vi "Write Multiple System Link Tags.vi"(7 "Force Initialize?":bool, 8 "error in (no error)":errorcluster, 9 "timestamp":timestamp, 10 "Values":dbl[](array[numeric]), 11 "SkyLine.Refs":refnum<class "NI Skyline Tag.lvclass">[](array[class])) -> (0 "error out":errorcluster)   [LabVIEW 2019, in "Data Publishing Service.lvlib"]
uses:
  Data Publishing Service.lvlib
  <vilib>/Skyline/Tag/Wrapper/Wrapper_class/NI Skyline Tag.lvclass
  <vilib>/Skyline/Tag/Wrapper/Wrapper_class/Tag Value Cluster Wrapper.ctl
  <vilib>/Skyline/Configuration/Configuration_class/NI Skyline Configuration.lvclass
  <vilib>/Skyline/Tag/Shared/typedefs/Tag Value Cluster.ctl
  <vilib>/Skyline/Tag/Shared/typedefs/DataType.ctl
  <vilib>/Skyline/Tag/Wrapper/Wrapper_class/Generate Tag Cluster (DBL) 2.vi
  <vilib>/Skyline/Tag/Shared/NI Skyline Tag.lvlib
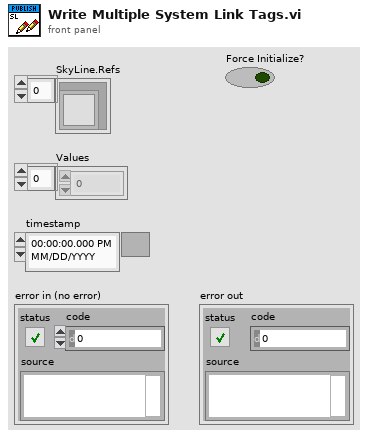
[diagram p1: front panel]
types:
  T1 = typedef "NI Skyline Tag.lvclass/Tag Value Cluster Wrapper.ctl" = cluster{"Configuration":refnum<class "NI Skyline Configuration.lvclass">, "Tag Cluster":T2}
  T2 = typedef "NI Skyline Tag.lvlib/Tag Value Cluster.ctl" = cluster{"Path":string, "Data Type":T3, "Value":string, "Time Stamp":timestamp}
  T3 = typedef "NI Skyline Tag.lvlib/DataType.ctl" = enum32{"Double", "I32", "String", "Boolean", "U64", "Timestamp"}
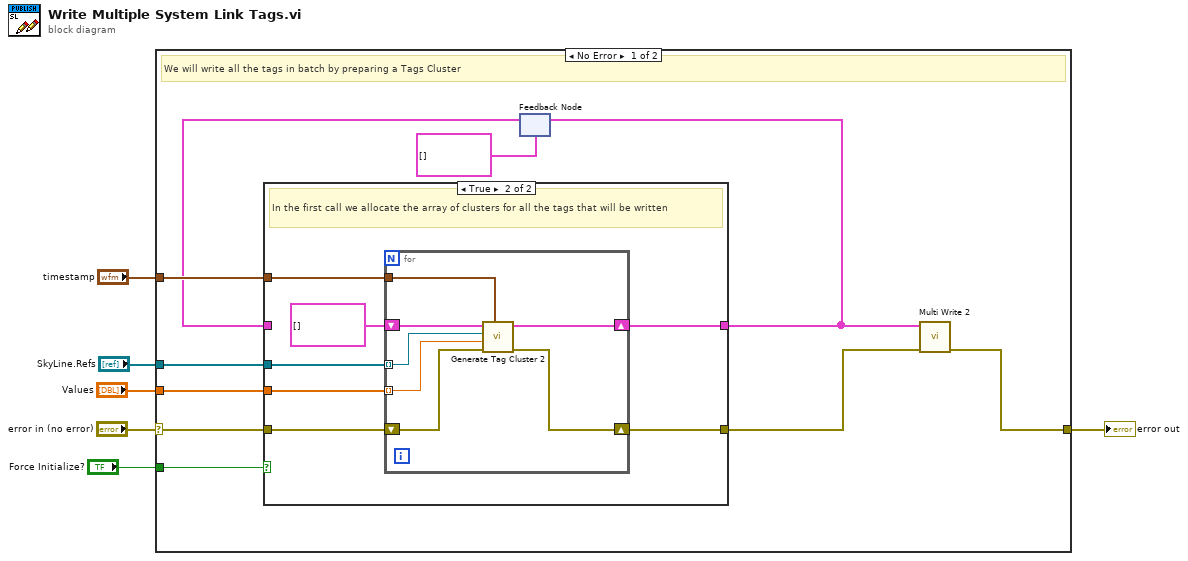
[diagram p0: block diagram]
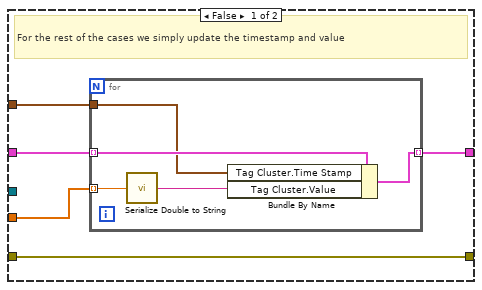
[diagram p2: hidden frame]
diagram:
  n1 = case shown="No Error" "error in (no error)" {
    selector: "error in (no error)" -> [w9 w41]
    tunnel: "SkyLine.Refs" -> [w16 _]
    tunnel: "Values" -> [w15 _]
    tunnel: "timestamp" -> [w14 _]
    tunnel: [w8 w41] -> w2
    tunnel: "Force Initialize?" -> [w7 _]
    frame No Error {
      # "We will write all the tags in batch by preparing a Tags Cluster"
      n2 = feedback #1(T1[] [] ("tag clusters in")) -> (w12:T1[])
      n3 = case shown="True" w7 {
        tunnel: w16 -> [_ w33]
        tunnel: w15 -> [w17 w32]
        tunnel: w9 -> [w21 w31]
        tunnel: w14 -> [w18 w30]
        tunnel: [w21 w29] -> w10
        tunnel: [w19 w28] -> w11
        tunnel: w12 -> [w20 _]
        frame False {
          # "For the rest of the cases we simply update the timestamp and value"
          n4 = for {
            tunnel: w20 -> [w26] mode=indexing
            tunnel: [w25] -> w19 mode=indexing
            tunnel: w18 -> [w24]
            tunnel: w17 -> [w22] mode=indexing
            n5 = call <vilib>:"Serialize Double to String.vi"("double"=w22) -> ("string"=w23:string)
            n6 = Bundle By Name(cluster=w26, "Tag Cluster.Time Stamp"=w24, "Tag Cluster.Value"=w23) -> (w25:T1)
          }
        }
        frame True {
          # "In the first call we allocate the array of clusters for all the tags that will be written"
          n7 = for {
            shift-right: [w36] -> w28
            shift-left: T1[] [] ("tag clusters in") -> [w40]
            tunnel: w33 -> [w39] mode=indexing
            tunnel: w32 -> [w38] mode=indexing
            shift-right: [w34] -> w29
            shift-left: w31 -> [w37]
            tunnel: w30 -> [w35]
            n8 = call-poly <vilib>:"Generate Tag Cluster 2.vi"("time stamp"=w35, "error in (no error)"=w37, "value"=w38, "tag in"=w39, "tag clusters in"=w40) -> ("error out"=w34:errorcluster, "tag clusters out"=w36:T1[])  [unwired: 4 in, 1 out]
          }
        }
      }
      n9 = feedback-in #1(w11) -> ()
      n10 = call <vilib>:"Multi Write 2.vi"("error in (no error)"=w10, "tag clusters"=w11) -> ("error out"=w8:errorcluster)  [unwired: 9 in]
    }
    frame Error {
    }
  }
  "error out" <- w2
